vi "Estado_posicion_sensores.vi"() -> ()   [LabVIEW 2020]
panel:
  out "Posicion sensores":T1
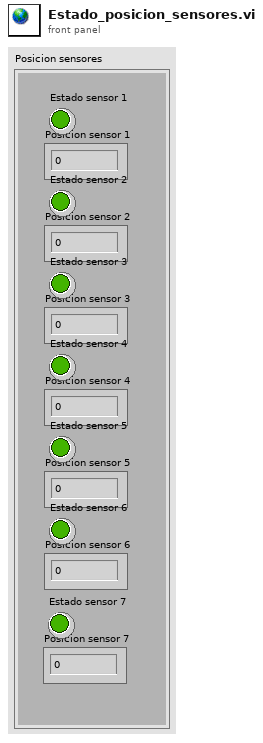
[diagram p1: front panel]
types:
  T1 = cluster{"Posicion sensor 1":i32, "Posicion sensor 2":i32, "Posicion sensor 3":i32, "Posicion sensor 4":i32, "Posicion sensor 5":i32, "Posicion sensor 6":i32, "Estado sensor 1":bool, "Estado sensor 2":bool, "Estado sensor 3":bool, "Estado sensor 4":bool, "Estado sensor 5":bool, "Estado sensor 6":bool, "Posicion sensor 7":i32, "Estado sensor 7":bool}
diagram:
